vi "Read Analogue.vi"(8 "error in (no error)":errorcluster, 11 "Lambda Gen Plus in":refnum<class "Lambda Gen Plus.lvclass">) -> (0 "error out":errorcluster, 2 "Waveforms":waveform(dbl)[](array[waveform]), 3 "Lambda Gen Plus out":refnum<class "Lambda Gen Plus.lvclass">)   [LabVIEW 2025, in "Power Supply.lvlib" / "Lambda Gen Plus.lvclass"]
uses:
  Lambda Gen Plus.lvclass
  C:/Users/Public/Documents/Sandia National Labs/TSS Plugin/Abstract Engine.lvlibp/Abstract Instrument/Abstract Instrument.lvclass
  Lambda Gen Plus.lvclass/Lambda Gen Plus.ctl
  <instrlib>/TDK-Lambda G Series/TDK-Lambda G Series.lvlib
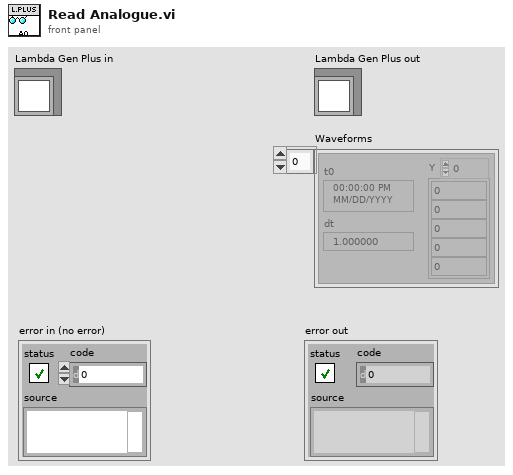
[diagram p1: front panel]
types:
  T1 = typedef "Abstract Engine.lvlibp/Abstract Instrument.lvclass/Channel.ctl" = cluster{"Alias":string, "DataType":enum16{"Anaolg Input", "Waveform"}, "Unit":enum16{"---", "V", "A", "Ohm", "Hz", "uF", "degC", "deg"}, "Upper limit":dbl, "Lower limit":dbl, "Measurement":variant}
  T2 = cluster{"Output Voltage (V)":dbl, "Output Current (A)":dbl}
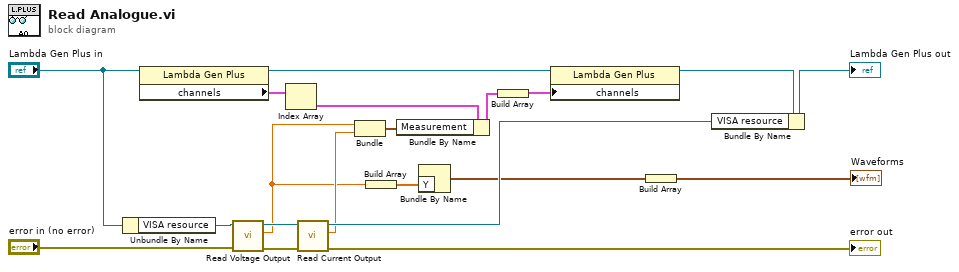
[diagram p0: block diagram]
diagram:
  n1 = Unbundle By Name("Lambda Gen Plus in") -> ("VISA resource"=w19:refnum<visa-resource-name>)
  n2 = property class="Lambda Gen Plus"(reference="Lambda Gen Plus in") -> (reference out=w12:refnum<class "Lambda Gen Plus.lvclass">, "channels"=w11:T1[])  [unwired: 1 in, 1 out]
  n3 = call <instrlib>:"Read Voltage Output.vi"("error in (no error)"="error in (no error)", "VISA resource name"=w19) -> ("error out"=w14:errorcluster, "Output Voltage (V)"=w4:dbl, "VISA resource name out"=w16:refnum<visa-resource-name>)  [unwired: 7 in]
  n4 = Index Array(array=w11) -> (element=w9:T1)  [unwired: 1 in]
  n5 = call <instrlib>:"Read Current Output.vi"("error in (no error)"=w14, "VISA resource name"=w16) -> ("error out"=→"error out":errorcluster, "Output Current (A)"=w8:dbl, "VISA resource name out"=w15:refnum<visa-resource-name>)  [unwired: 7 in]
  n6 = Bundle("Output Voltage (V)"=w4, "Output Current (A)"=w8) -> (w10:T2)  [unwired: 1 in]
  n7 = Build Array(w4) -> (w3:dbl[])
  n8 = Bundle By Name(cluster=w9, "Measurement"=w10) -> (w6:T1)
  n9 = Bundle By Name("Y"=w3) -> (w2:waveform(dbl))  [unwired: 1 in]
  n10 = Build Array(w6) -> (w7:T1[])
  n11 = property class="Lambda Gen Plus"(reference=w12, "channels"=w7) -> (reference out=w17:refnum<class "Lambda Gen Plus.lvclass">)  [unwired: 1 in, 1 out]
  n12 = Build Array(w2) -> (→"Waveforms":waveform(dbl)[])
  n13 = Bundle By Name(cluster=w17, "VISA resource"=w15) -> (→"Lambda Gen Plus out":refnum<class "Lambda Gen Plus.lvclass">)
